vi "Jeff K one Line.vi"() -> ()   [LabVIEW 2025]
uses:
  <vilib>/Analysis/2dsp.llb/Complex FFT.vi
  <vilib>/Analysis/1siggen.llb/Ramp Pattern by Samples.vi
  <extravilib>/ChannelInstances/Tag-cdb/Instantiate.vi
  <extravilib>/ChannelInstances/Tag-cdb/EndpointRead.vi
  <extravilib>/ChannelInstances/Tag-cdb/Endpoint.vi
  <vilib>/Analysis/NI_AALPro.lvlib
  <vilib>/Analysis/NI_AALBase.lvlib
  <vilib>/Analysis/2dsp.llb/Resample (constant to constant, complex single-channel).vi
  <extravilib>/ChannelInstances/Tag-cdb.lvlib
panel:
  out "XY Graph 2":cluster{"XY Graph - Light":cdb[]}[](graph)
  out "XY Graph":cluster{"XY Graph - Light":cdb[]}[](graph)
  in  "index":i32=30
  in  "Individual Plots Per Vector":bool=TRUE
  in  "milliseconds to wait":u32=70
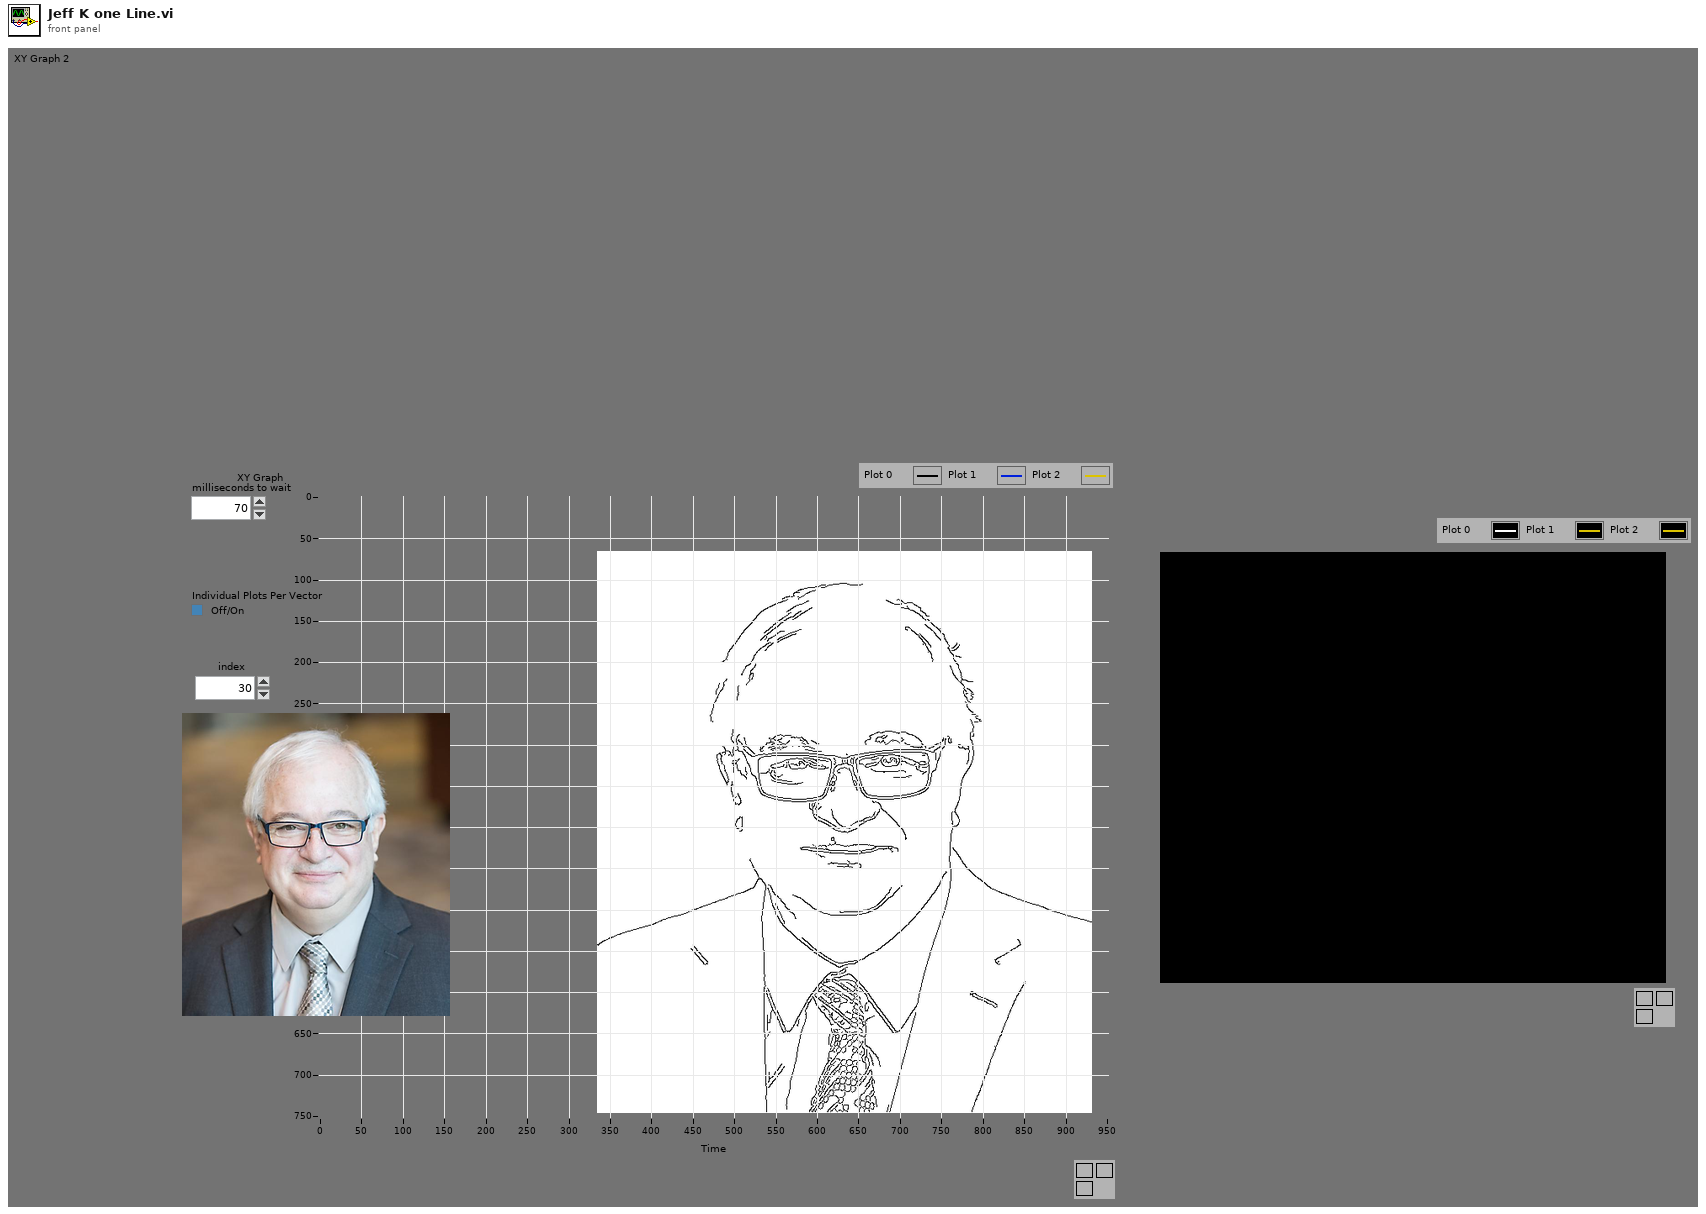
[diagram p1: front panel]
types:
  T1 = typedef "Tag-cdb.lvlib/))Channel.ctl" = refnum<queue>
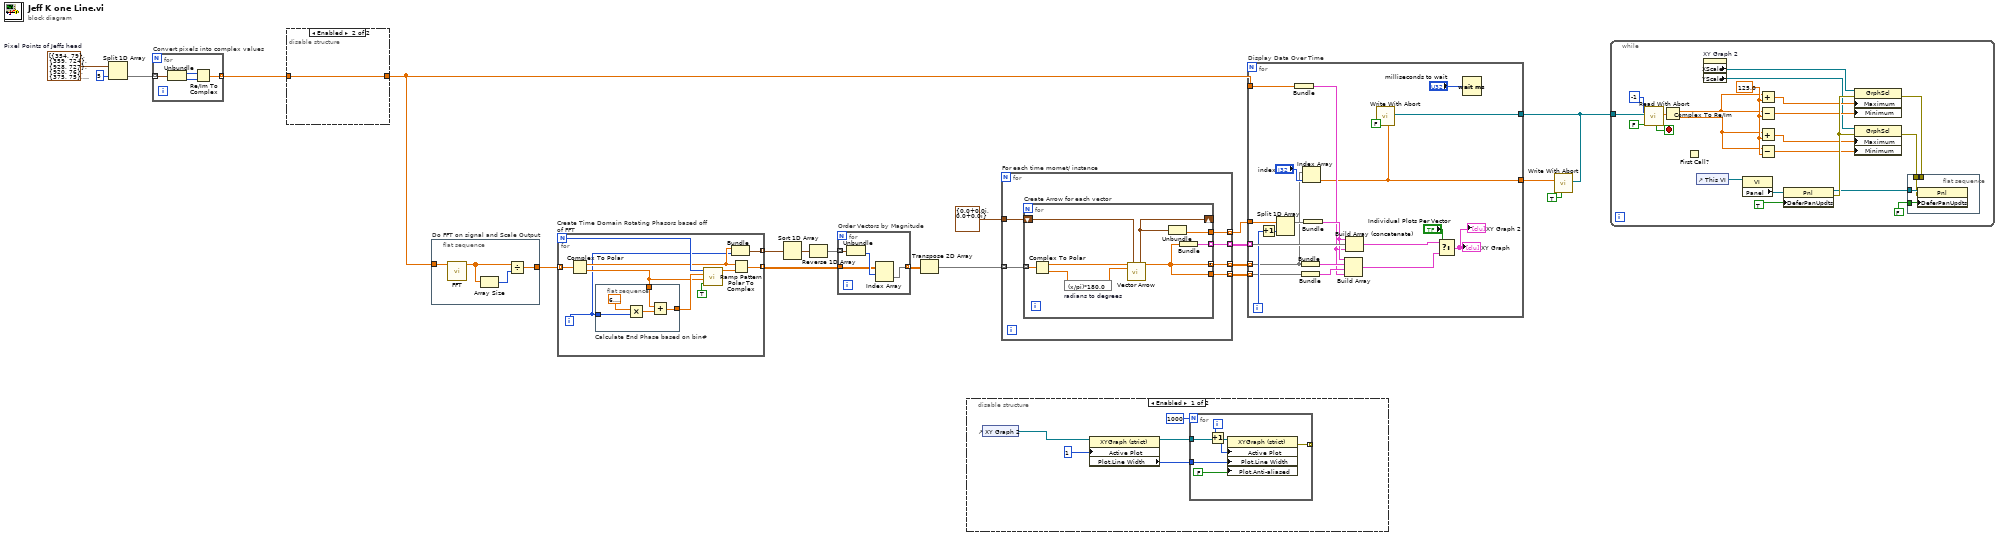
[diagram p0: block diagram]
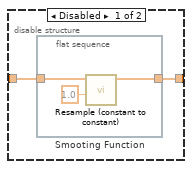
[diagram p2: hidden frame]
diagram:
  w13 = cluster{"Horizontal":i32, "Vertical":i32}[] [{"Horizontal"=354, "Vertical"=79}, {"Horizontal"=359, "Vertical"=724}, {"Horizontal"=928, "Vertical"=727}, {"Horizontal"=920, "Vertical"=76}, {"Horizontal"=375, "Vertical"=75}, {"Horizontal"=348, "Vertical"=534}, {"Horizontal"=379, "Vertical"=519}, {"Horizontal"=407, "Vertical"=510}, {"Horizontal"=436, "Vertical"=501}, {"Horizontal"=463, "Vertical"=490}, {"Horizontal"=491, "Vertical"=484}, {"Horizontal"=514, "Vertical"=473}, {"Horizontal"=528, "Vertical"=466}, {"Horizontal"=536, "Vertical"=452}, {"Horizontal"=523, "Vertical"=437}, {"Horizontal"=518, "Vertical"=417}, {"Horizontal"=512, "Vertical"=396}, {"Horizontal"=508, "Vertical"=372}, {"Horizontal"=503, "Vertical"=348}, {"Horizontal"=490, "Vertical"=331}, {"Horizontal"=491, "Vertical"=315}, {"Horizontal"=502, "Vertical"=290}, {"Horizontal"=511, "Vertical"=302}, {"Horizontal"=520, "Vertical"=312}, {"Horizontal"=529, "Vertical"=324}, {"Horizontal"=531, "Vertical"=338}, {"Horizontal"=536, "Vertical"=353}, {"Horizontal"=547, "Vertical"=354}, {"Horizontal"=563, "Vertical"=359}, {"Horizontal"=570, "Vertical"=361}, {"Horizontal"=586, "Vertical"=363}, {"Horizontal"=595, "Vertical"=363}, {"Horizontal"=610, "Vertical"=363}, {"Horizontal"=617, "Vertical"=349}, {"Horizontal"=623, "Vertical"=335}, {"Horizontal"=629, "Vertical"=318}, {"Horizontal"=618, "Vertical"=309}, {"Horizontal"=601, "Vertical"=306}, {"Horizontal"=587, "Vertical"=303}, {"Horizontal"=567, "Vertical"=299}, {"Horizontal"=551, "Vertical"=301}, {"Horizontal"=539, "Vertical"=305}, {"Horizontal"=529, "Vertical"=306}, {"Horizontal"=520, "Vertical"=296}, {"Horizontal"=512, "Vertical"=281}, {"Horizontal"=506, "Vertical"=277}, {"Horizontal"=502, "Vertical"=269}, {"Horizontal"=508, "Vertical"=250}, {"Horizontal"=516, "Vertical"=232}, {"Horizontal"=525, "Vertical"=213}, {"Horizontal"=539, "Vertical"=188}, {"Horizontal"=547, "Vertical"=174}, {"Horizontal"=563, "Vertical"=162}, {"Horizontal"=579, "Vertical"=144}, {"Horizontal"=587, "Vertical"=136}, {"Horizontal"=610, "Vertical"=128}, {"Horizontal"=629, "Vertical"=129}, {"Horizontal"=656, "Vertical"=127}, {"Horizontal"=666, "Vertical"=131}, {"Horizontal"=697, "Vertical"=140}, {"Horizontal"=711, "Vertical"=143}, {"Horizontal"=745, "Vertical"=163}, {"Horizontal"=750, "Vertical"=169}, {"Horizontal"=757, "Vertical"=193}, {"Horizontal"=771, "Vertical"=200}, {"Horizontal"=767, "Vertical"=224}, {"Horizontal"=774, "Vertical"=238}, {"Horizontal"=779, "Vertical"=268}, {"Horizontal"=783, "Vertical"=284}, {"Horizontal"=765, "Vertical"=286}, {"Horizontal"=746, "Vertical"=291}, {"Horizontal"=737, "Vertical"=300}, {"Horizontal"=718, "Vertical"=302}, {"Horizontal"=696, "Vertical"=299}, {"Horizontal"=679, "Vertical"=302}, {"Horizontal"=655, "Vertical"=304}, {"Horizontal"=650, "Vertical"=306}, {"Horizontal"=636, "Vertical"=308}, {"Horizontal"=620, "Vertical"=309}, {"Horizontal"=643, "Vertical"=317}, {"Horizontal"=651, "Vertical"=334}, {"Horizontal"=656, "Vertical"=342}, {"Horizontal"=664, "Vertical"=358}, {"Horizontal"=674, "Vertical"=367}, {"Horizontal"=689, "Vertical"=360}, {"Horizontal"=712, "Vertical"=361}, {"Horizontal"=731, "Vertical"=353}, {"Horizontal"=738, "Vertical"=346}, {"Horizontal"=747, "Vertical"=326}, {"Horizontal"=744, "Vertical"=315}, {"Horizontal"=751, "Vertical"=304}, {"Horizontal"=759, "Vertical"=294}, {"Horizontal"=773, "Vertical"=291}, {"Horizontal"=785, "Vertical"=286}, {"Horizontal"=770, "Vertical"=296}, {"Horizontal"=778, "Vertical"=306}, {"Horizontal"=776, "Vertical"=317}, {"Horizontal"=775, "Vertical"=326}, {"Horizontal"=773, "Vertical"=340}, {"Horizontal"=771, "Vertical"=353}, {"Horizontal"=765, "Vertical"=360}, {"Horizontal"=762, "Vertical"=383}, {"Horizontal"=763, "Vertical"=406}, {"Horizontal"=761, "Vertical"=420}, {"Horizontal"=778, "Vertical"=434}, {"Horizontal"=782, "Vertical"=446}, {"Horizontal"=798, "Vertical"=459}, {"Horizontal"=811, "Vertical"=468}, {"Horizontal"=829, "Vertical"=476}, {"Horizontal"=847, "Vertical"=485}, {"Horizontal"=865, "Vertical"=489}, {"Horizontal"=878, "Vertical"=495}, {"Horizontal"=891, "Vertical"=500}, {"Horizontal"=903, "Vertical"=505}, {"Horizontal"=926, "Vertical"=511}, {"Horizontal"=912, "Vertical"=713}, {"Horizontal"=794, "Vertical"=706}, {"Horizontal"=812, "Vertical"=684}, {"Horizontal"=820, "Vertical"=665}, {"Horizontal"=829, "Vertical"=650}, {"Horizontal"=835, "Vertical"=631}, {"Horizontal"=844, "Vertical"=612}, {"Horizontal"=853, "Vertical"=594}, {"Horizontal"=859, "Vertical"=579}, {"Horizontal"=851, "Vertical"=571}, {"Horizontal"=840, "Vertical"=563}, {"Horizontal"=827, "Vertical"=556}, {"Horizontal"=837, "Vertical"=547}, {"Horizontal"=849, "Vertical"=536}, {"Horizontal"=851, "Vertical"=528}, {"Horizontal"=844, "Vertical"=519}, {"Horizontal"=840, "Vertical"=498}, {"Horizontal"=832, "Vertical"=485}, {"Horizontal"=829, "Vertical"=473}, {"Horizontal"=758, "Vertical"=419}, {"Horizontal"=760, "Vertical"=437}, {"Horizontal"=762, "Vertical"=465}, {"Horizontal"=755, "Vertical"=482}, {"Horizontal"=751, "Vertical"=506}, {"Horizontal"=744, "Vertical"=525}, {"Horizontal"=739, "Vertical"=547}, {"Horizontal"=731, "Vertical"=561}, {"Horizontal"=726, "Vertical"=580}, {"Horizontal"=723, "Vertical"=604}, {"Horizontal"=719, "Vertical"=620}, {"Horizontal"=715, "Vertical"=637}, {"Horizontal"=706, "Vertical"=665}, {"Horizontal"=705, "Vertical"=683}, {"Horizontal"=701, "Vertical"=700}, {"Horizontal"=698, "Vertical"=709}, {"Horizontal"=694, "Vertical"=718}, {"Horizontal"=689, "Vertical"=722}, {"Horizontal"=676, "Vertical"=712}, {"Horizontal"=674, "Vertical"=695}, {"Horizontal"=667, "Vertical"=682}, {"Horizontal"=671, "Vertical"=666}, {"Horizontal"=660, "Vertical"=646}, {"Horizontal"=664, "Vertical"=635}, {"Horizontal"=668, "Vertical"=624}, {"Horizontal"=675, "Vertical"=620}, {"Horizontal"=679, "Vertical"=623}, {"Horizontal"=692, "Vertical"=630}, {"Horizontal"=693, "Vertical"=633}, {"Horizontal"=698, "Vertical"=635}, {"Horizontal"=711, "Vertical"=628}, {"Horizontal"=721, "Vertical"=615}, {"Horizontal"=726, "Vertical"=586}, {"Horizontal"=746, "Vertical"=531}, {"Horizontal"=758, "Vertical"=482}, {"Horizontal"=753, "Vertical"=456}, {"Horizontal"=740, "Vertical"=475}, {"Horizontal"=727, "Vertical"=490}, {"Horizontal"=713, "Vertical"=503}, {"Horizontal"=696, "Vertical"=531}, {"Horizontal"=683, "Vertical"=529}, {"Horizontal"=671, "Vertical"=538}, {"Horizontal"=659, "Vertical"=550}, {"Horizontal"=642, "Vertical"=552}, {"Horizontal"=628, "Vertical"=553}, {"Horizontal"=602, "Vertical"=550}, {"Horizontal"=592, "Vertical"=529}, {"Horizontal"=586, "Vertical"=528}, {"Horizontal"=579, "Vertical"=519}, {"Horizontal"=570, "Vertical"=508}, {"Horizontal"=564, "Vertical"=492}, {"Horizontal"=557, "Vertical"=481}, {"Horizontal"=553, "Vertical"=470}, {"Horizontal"=548, "Vertical"=456}, {"Horizontal"=540, "Vertical"=468}, {"Horizontal"=541, "Vertical"=485}, {"Horizontal"=542, "Vertical"=508}, {"Horizontal"=539, "Vertical"=527}, {"Horizontal"=544, "Vertical"=555}, {"Horizontal"=543, "Vertical"=588}, {"Horizontal"=539, "Vertical"=614}, {"Horizontal"=539, "Vertical"=631}, {"Horizontal"=539, "Vertical"=656}, {"Horizontal"=542, "Vertical"=673}, {"Horizontal"=539, "Vertical"=687}, {"Horizontal"=545, "Vertical"=712}, {"Horizontal"=542, "Vertical"=723}, {"Horizontal"=547, "Vertical"=727}, {"Horizontal"=572, "Vertical"=724}, {"Horizontal"=578, "Vertical"=696}, {"Horizontal"=578, "Vertical"=682}, {"Horizontal"=586, "Vertical"=659}, {"Horizontal"=588, "Vertical"=638}, {"Horizontal"=593, "Vertical"=613}, {"Horizontal"=601, "Vertical"=601}, {"Horizontal"=609, "Vertical"=614}, {"Horizontal"=613, "Vertical"=626}, {"Horizontal"=625, "Vertical"=640}, {"Horizontal"=614, "Vertical"=670}, {"Horizontal"=610, "Vertical"=680}, {"Horizontal"=604, "Vertical"=701}, {"Horizontal"=604, "Vertical"=706}, {"Horizontal"=602, "Vertical"=710}, {"Horizontal"=597, "Vertical"=718}, {"Horizontal"=596, "Vertical"=718}, {"Horizontal"=597, "Vertical"=718}, {"Horizontal"=596, "Vertical"=717}, {"Horizontal"=596, "Vertical"=717}, {"Horizontal"=597, "Vertical"=715}, {"Horizontal"=598, "Vertical"=709}, {"Horizontal"=598, "Vertical"=709}, {"Horizontal"=597, "Vertical"=709}, {"Horizontal"=573, "Vertical"=709}, {"Horizontal"=585, "Vertical"=684}, {"Horizontal"=591, "Vertical"=655}, {"Horizontal"=597, "Vertical"=623}, {"Horizontal"=599, "Vertical"=596}, {"Horizontal"=588, "Vertical"=609}, {"Horizontal"=577, "Vertical"=631}, {"Horizontal"=566, "Vertical"=639}, {"Horizontal"=539, "Vertical"=591}, {"Horizontal"=545, "Vertical"=484}, {"Horizontal"=563, "Vertical"=510}, {"Horizontal"=582, "Vertical"=478}, {"Horizontal"=595, "Vertical"=486}, {"Horizontal"=606, "Vertical"=492}, {"Horizontal"=641, "Vertical"=500}, {"Horizontal"=652, "Vertical"=495}, {"Horizontal"=660, "Vertical"=496}, {"Horizontal"=684, "Vertical"=488}, {"Horizontal"=695, "Vertical"=478}, {"Horizontal"=701, "Vertical"=471}, {"Horizontal"=695, "Vertical"=427}, {"Horizontal"=683, "Vertical"=432}, {"Horizontal"=660, "Vertical"=437}, {"Horizontal"=651, "Vertical"=441}, {"Horizontal"=635, "Vertical"=438}, {"Horizontal"=615, "Vertical"=436}, {"Horizontal"=605, "Vertical"=434}, {"Horizontal"=594, "Vertical"=429}, {"Horizontal"=587, "Vertical"=422}, {"Horizontal"=591, "Vertical"=415}, {"Horizontal"=603, "Vertical"=422}, {"Horizontal"=619, "Vertical"=424}, {"Horizontal"=629, "Vertical"=424}, {"Horizontal"=645, "Vertical"=423}, {"Horizontal"=653, "Vertical"=422}, {"Horizontal"=661, "Vertical"=422}, {"Horizontal"=679, "Vertical"=421}, {"Horizontal"=686, "Vertical"=419}, {"Horizontal"=687, "Vertical"=418}, {"Horizontal"=705, "Vertical"=409}, {"Horizontal"=696, "Vertical"=390}, {"Horizontal"=687, "Vertical"=382}, {"Horizontal"=676, "Vertical"=378}, {"Horizontal"=664, "Vertical"=386}, {"Horizontal"=648, "Vertical"=397}, {"Horizontal"=642, "Vertical"=397}, {"Horizontal"=626, "Vertical"=394}, {"Horizontal"=616, "Vertical"=389}, {"Horizontal"=605, "Vertical"=383}, {"Horizontal"=606, "Vertical"=375}, {"Horizontal"=616, "Vertical"=361}, {"Horizontal"=624, "Vertical"=344}, {"Horizontal"=631, "Vertical"=329}, {"Horizontal"=641, "Vertical"=322}, {"Horizontal"=648, "Vertical"=330}, {"Horizontal"=657, "Vertical"=349}, {"Horizontal"=669, "Vertical"=360}, {"Horizontal"=681, "Vertical"=369}]  # Pixel Points of Jeffs head
  n1 = Split 1D Array(array=w13, index=5) -> (second subarray=w12:cluster{"Horizontal":i32, "Vertical":i32}[])  [unwired: 1 out]
  n2 = for "Convert pixels into complex values" {
    tunnel: w12 -> [w24] mode=indexing
    tunnel: [w21] -> w18 mode=indexing
    n3 = Unbundle(w24) -> ("Horizontal"=w23:i32, "Vertical"=w22:i32)
    n4 = Re/Im To Complex(1:w22, 2:w23) -> (0:w21:cdb)
  }
  n5 = disable-structure shown="Enabled" {
    disable-tunnel: w18 -> [w26 w30]
    disable-tunnel: [w25 w30] -> w14
    frame Disabled {
      n6 = flat-sequence "Smooting Function" {
        tunnel: w26 -> [w29]
        tunnel: [w27] -> w25
        frame #0 {
          n7 = call-poly <vilib>:"Resample (constant to constant).vi"("dt"=1.0, "X"=w29) -> ("Y"=w27:cdb[])  [unwired: 7 in, 2 out]
        }
      }
    }
    frame Enabled {
    }
  }
  n8 = flat-sequence "Do FFT on signal and Scale Output" {
    tunnel: [w33] -> w9
    tunnel: w14 -> [w32]
    frame #0 {
      n9 = call-poly <vilib>:"FFT.vi"("X"=w32) -> ("FFT {X}"=w34:cdb[])  [unwired: 9 in, 1 out]
      n10 = Array Size(array=w34) -> (size(s)=w31:i32)
      n11 = Divide(x=w34, y=w31) -> (x/y=w33:cdb[])
    }
  }
  n12 = for "Create Time Domain Rotating Phasors based off of FFT" {
    N -> [w42]
    tunnel: w9 -> [w44] mode=indexing
    tunnel: [w40] -> w6 mode=indexing
    tunnel: [w35] -> w8 mode=indexing
    i -> [w36]
    n13 = Complex To Polar(r * e^(i*theta)=w44) -> (r=w37:dbl, theta=w38:dbl)
    n14 = flat-sequence "Calculate End Phase based on bin#" {
      tunnel: [w47] -> w43
      tunnel: w36 -> [w46]
      tunnel: w38 -> [w45]
      frame #0 {
        n15 = Multiply(x=6.283185307179586, y=w46) -> (x*y=w48:dbl)
        n16 = Add(x=w45, y=w48) -> (x+y=w47:dbl)
      }
    }
    n17 = call-poly <vilib>:"Ramp Pattern.vi"("exclude end?"=TRUE, "start"=w38, "end"=w43, "samples"=w42) -> ("Ramp Pattern"=w41:dbl[])  [unwired: 6 in, 1 out]
    n18 = Bundle(w37, w36) -> (w35:cluster{dbl, i32})  [unwired: 1 in]
    n19 = Polar To Complex(1:w41, 2:w37) -> (0:w40:cdb[])
  }
  n20 = Sort 1D Array(array=w8) -> (sorted array=w7:cluster{dbl, i32}[])
  n21 = Reverse 1D Array(array=w7) -> (reversed array=w4:cluster{dbl, i32}[])
  n22 = for "Order Vectors by Magnitude" {
    tunnel: w4 -> [w53] mode=indexing
    tunnel: w6 -> [w51]
    tunnel: [w50] -> w5 mode=indexing
    n23 = Unbundle(w53) -> (w52:i32)  [unwired: 1 out]
    n24 = Index Array(array=w51, index (row)=w52) -> (element=w50:cdb[])  [unwired: 1 in]
  }
  n25 = Transpose 2D Array(2D array=w5) -> (transposed array=w19:cdb[][])
  n26 = disable-structure shown="Enabled" {
    frame Enabled {
      n27 = control-ref of="XY Graph 2"() -> (w54:refnum<vi>)
      n28 = property class="XYGraph (strict)"(reference=w54, "Active Plot"=u32 1) -> (reference out=w57:refnum<vi>, "Plot.Line Width"=w55:u8)  [unwired: 1 in, 1 out]
      n29 = for {
        N: 1000 -> [_]
        tunnel: w57 -> [w64]
        tunnel: [w63] -> _ mode=indexing
        tunnel: w55 -> [w61]
        i -> [w62]
        n30 = Increment(x=w62) -> (x+1=w59:i32)
        n31 = property class="XYGraph (strict)"(reference=w64, "Active Plot"=w59, "Plot.Line Width"=w61, "Plot.Anti-aliased"=FALSE) -> (error out=w63:errorcluster)  [unwired: 1 in, 1 out]
      }
    }
    frame Disabled {
    }
  }
  n32 = for "For each time momet/ instance" {
    tunnel: cluster{"Initial":cdb, "Endpoint":cdb} {"Initial"=0.0+0.0i, "Endpoint"=0.0+0.0i} ("Resultant Vector") -> [w70]
    tunnel: w19 -> [w68] mode=indexing
    tunnel: [w69] -> w17 mode=indexing
    tunnel: [w67] -> w16 mode=indexing
    tunnel: [w66] -> w15 mode=indexing
    tunnel: [w65] -> w10 mode=indexing
    n33 = for "Create Arrow for each vector" {
      tunnel: [w79] -> w69 mode=indexing
      shift-right: [w72] -> _
      shift-left: w70 -> [w78]
      tunnel: w68 -> [w77] mode=indexing
      tunnel: [w76] -> w67 mode=concatenating
      tunnel: [w76] -> w66
      tunnel: [w71] -> w65
      n34 = Complex To Polar(r * e^(i*theta)=w77) -> (r=w75:dbl, theta=w74:dbl)
      n35 = expression code="(x/pi)*180.0" "radians to degrees"(w74) -> (w73:dbl)
      n36 = call "Vector Arrow.vi"("Magnitude"=w75, "Initial Vector"=w78, "Phase, deg"=w73) -> ("Resultant Vector"=w72:cluster{"Initial":cdb, "Endpoint":cdb}, "XY Graph - Light"=w76:cdb[])  [unwired: 11 in]
      n37 = Unbundle(w72) -> ("Endpoint"=w71:cdb)  [unwired: 1 out]
      n38 = Bundle("XY Graph - Light"=w76) -> (w79:cluster{"XY Graph - Light":cdb[]})  [unwired: 1 in]
    }
  }
  n39 = for "Display Data Over Time" {
    tunnel: w17 -> [w96] mode=indexing
    tunnel: w16 -> [w80] mode=indexing
    tunnel: w14 -> [w98]
    tunnel: w15 -> [w81] mode=indexing
    tunnel: w10 -> [w91]
    tunnel: [w85] -> w1
    tunnel: [w84] -> w3
    i -> [w90]
    n40 = Increment(x=w90) -> (x+1=w89:i32)
    n41 = Split 1D Array(array=w91, index=w89) -> (first subarray=w86:cdb[])  [unwired: 1 out]
    n42 = Bundle(w98) -> (w87:cluster{cdb[]})  [unwired: 1 in]
    n43 = Bundle("XY Graph - Light"=w80) -> (w99:cluster{"XY Graph - Light":cdb[]})  [unwired: 1 in]
    n44 = Bundle("XY Graph - Light"=w81) -> (w97:cluster{"XY Graph - Light":cdb[]})  [unwired: 1 in]
    n45 = Index Array(array=w80, index="index") -> (element=w84:cdb)
    n46 = Bundle(w86) -> (w88:cluster{cdb[]})  [unwired: 1 in]
    n47 = Build Array(w88, w99, w97, w87) -> (w94:cluster{"XY Graph - Light":cdb[]}[])
    n48 = Build Array (concatenate)(w88, w96, w87) -> (w95:cluster{"XY Graph - Light":cdb[]}[])
    n49 = call <extravilib>:"Write With Abort.vi"("abort"=FALSE, "element"=w84) -> ("channel"=w85:T1)  [unwired: 7 in, 2 out]
    n50 = Select(t=w95, s="Individual Plots Per Vector", f=w94) -> (s? t:f=→"XY Graph" →"XY Graph 2":cluster{"XY Graph - Light":cdb[]}[])
    n51 = Wait (ms)(milliseconds to wait="milliseconds to wait") -> ()  [unwired: 1 out]
  }
  n52 = call <extravilib>:"Write With Abort.vi"("channel"=w1, "abort"=TRUE, "element"=w3) -> ()  [unwired: 7 in, 2 out]
  n53 = while {
    tunnel: w1 -> [w114]
    stop <- w112 stop-if-true
    w115 = 125.0 ("y")
    n54 = call <extravilib>:"Read With Abort.vi"("abort"=FALSE, "timeout in ms (0)"=-1, "channel"=w114) -> ("element"=w113:cdb, "aborted?"=w112:bool)  [unwired: 6 in, 1 out]
    n55 = Complex To Re/Im(x + iy=w113) -> (x=w110:dbl, y=w109:dbl)
    n56 = First Call?() -> ()  [unwired: 1 out]
    n57 = control-ref of="This VI"() -> (w101:refnum<vi>)
    n58 = property on="XY Graph 2" class="XYGraph (strict)"() -> ("XScale"=w116:refnum<vi>, "YScale"=w117:refnum<vi>)  [unwired: 2 in, 2 out]
    n59 = property class="VI"(reference=w101) -> ("Panel"=w108:refnum<vi>)  [unwired: 1 in, 2 out]
    n60 = Add(x=w110, y=w115) -> (x+y=w121:dbl)
    n61 = Subtract(x=w110, y=w115) -> (x-y=w120:dbl)
    n62 = Add(x=w109, y=w115) -> (x+y=w119:dbl)
    n63 = Subtract(x=w109, y=w115) -> (x-y=w118:dbl)
    n64 = property class="Pnl"(reference=w108, "DeferPanUpdts"=TRUE ("Defer Panel Updates")) -> (reference out=w106:refnum<vi>, error out=w122:errorcluster)  [unwired: 1 in]
    n65 = property class="GrphScl"(reference=w116, error in=w122, "Maximum"=w121, "Minimum"=w120) -> (error out=w104:errorcluster)  [unwired: 1 out]
    n66 = property class="GrphScl"(reference=w117, error in=w122, "Maximum"=w119, "Minimum"=w118) -> (error out=w105:errorcluster)  [unwired: 1 out]
    n67 = flat-sequence {
      tunnel: w106 -> [w125]
      tunnel: w105 -> [w124]
      tunnel: w104 -> [_]
      tunnel: FALSE ("DeferPanUpdts") -> [w123]
      frame #0 {
        n68 = property class="Pnl"(reference=w125, error in=w124, "DeferPanUpdts"=w123) -> ()  [unwired: 2 out]
      }
    }
  }
